vi "XBEE Close.vi"(0 "error in (no error)":errorcluster, 1 "VISA resource name":refnum<visa-resource-name>) -> ()   [LabVIEW 2012]
doc: "This VI will close the port used to communicate using an XBee."
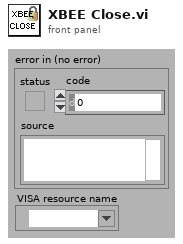
[diagram p1: front panel]
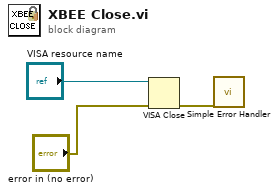
[diagram p0: block diagram]
diagram:
  n1 = VISA Close(VISA resource name="VISA resource name", error in (no error)="error in (no error)") -> (error out=w3:errorcluster)
  n2 = call <vilib>:"Simple Error Handler.vi"("error in (no error)"=w3) -> ()  [unwired: 1 in, 8 out]
